vi "保存程序.vi"(8 "error in (no error)":errorcluster caption="错误输入（无错误）", 11 "程序 输入":refnum<class "程序.lvclass">) -> (0 "error out":errorcluster caption="错误输出", 3 "程序 输出":refnum<class "程序.lvclass">)   [LabVIEW 2020, in "程序.lvclass"]
uses:
  D:/SuperPython-master/ScintillaNET.dll
  ScintillaNET.dll
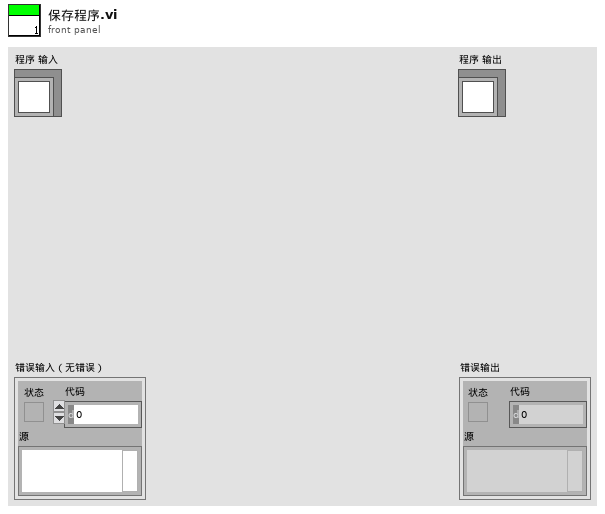
[diagram p1: front panel]
types:
  T1 = enum16{"open", "replace", "create", "open or create", "replace or create", "replace or create with confirmation"}
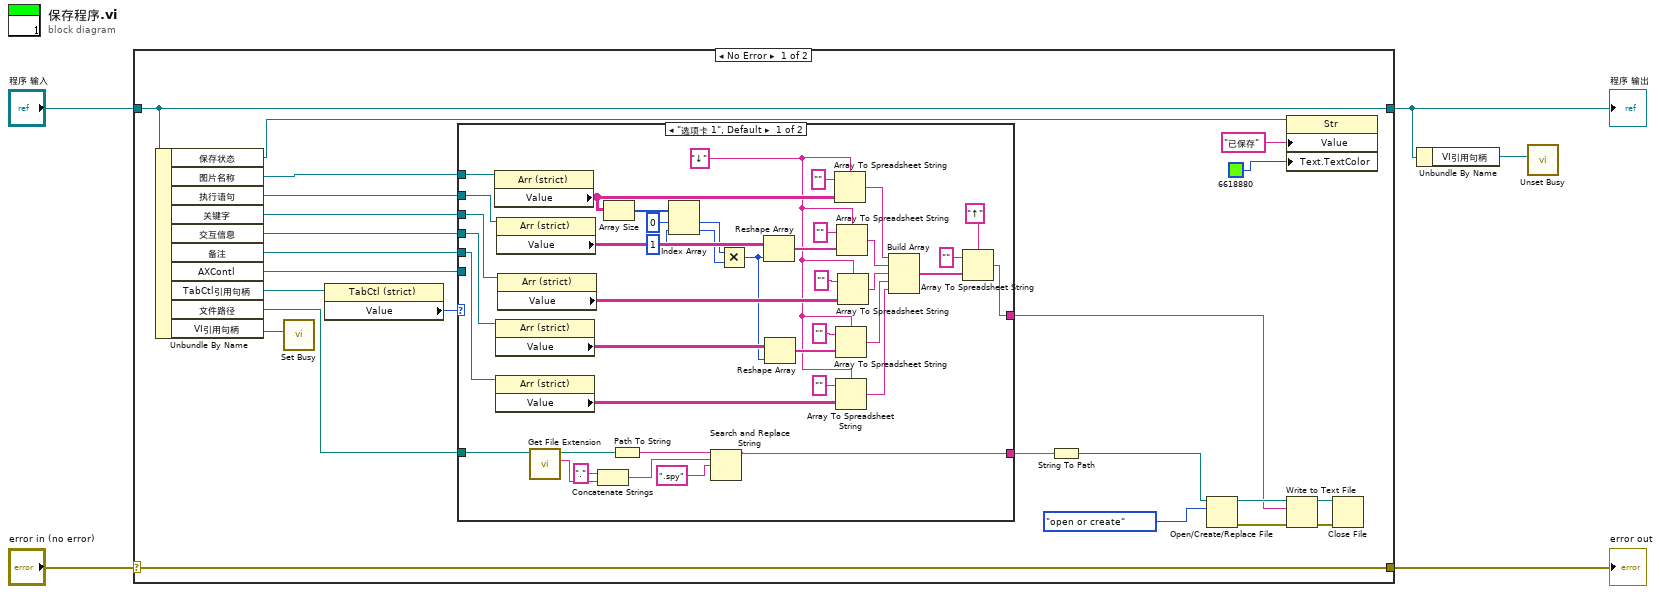
[diagram p0: block diagram]
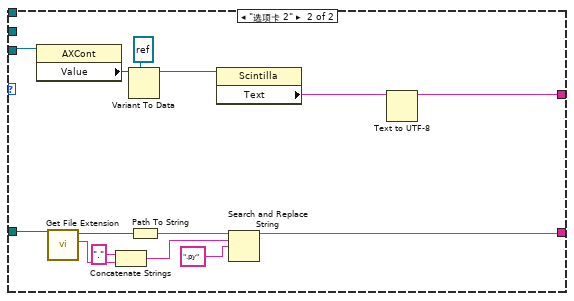
[diagram p2: hidden frame]
diagram:
  n1 = case shown="No Error" "error in (no error)" {
    selector: "error in (no error)" -> [w28 w85]
    tunnel: [w28 w85] -> w4
    tunnel: [w22 w84] -> w2
    tunnel: "程序 输入" -> [w22 w84]
    frame No Error {
      n2 = Unbundle By Name(w22) -> ("保存状态"=w14:refnum<vi>, "图片名称"=w21:refnum<vi>, "执行语句"=w20:refnum<vi>, "关键字"=w19:refnum<vi>, "交互信息"=w17:refnum<vi>, "备注"=w16:refnum<vi>, "AXContl"=w11:refnum<vi>, "TabCtl引用句柄"=w10:refnum<vi>, "文件路径"=w8:path, "VI引用句柄"=w12:refnum<vi>)
      n3 = call <vilib>:"Set Busy.vi"("VI reference (current VI)"=w12) -> ()  [unwired: 9 in, 2 out]
      n4 = property class="TabCtl (strict)"(reference=w10) -> ("Value"=w9:enum32{"选项卡 1", "选项卡 2"})  [unwired: 1 in, 2 out]
      n5 = case shown="\"选项卡 1\", Default" w9 {
        tunnel: [w68 w70] -> w23
        tunnel: w21 -> [w66 _]
        tunnel: w20 -> [w65 _]
        tunnel: w19 -> [w64 _]
        tunnel: w17 -> [w54 _]
        tunnel: w16 -> [w41 _]
        tunnel: w11 -> [_ w80]
        tunnel: w8 -> [w30 w79]
        tunnel: [w29 w73] -> w7
        frame "选项卡 1", Default {
          w38 = "↓" ("分隔符(Tab)")
          n6 = property class="Arr (strict)"(reference=w66) -> ("Value"=w48:string[][])  [unwired: 1 in, 2 out]
          n7 = property class="Arr (strict)"(reference=w54) -> ("Value"=w52:string[][])  [unwired: 1 in, 2 out]
          n8 = property class="Arr (strict)"(reference=w41) -> ("Value"=w40:string[][])  [unwired: 1 in, 2 out]
          n9 = property class="Arr (strict)"(reference=w65) -> ("Value"=w50:string[][])  [unwired: 1 in, 2 out]
          n10 = property class="Arr (strict)"(reference=w64) -> ("Value"=w60:string[][])  [unwired: 1 in, 2 out]
          n11 = call <vilib>:"Get File Extension.vi"("file"=w30) -> ("lowercase file extension"=w33:string, "dup file"=w36:path)  [unwired: 6 in, 3 out]
          n12 = Concatenate Strings("." ("字符串"), w33) -> (w32:string)
          n13 = Array Size(array=w48) -> (size(s)=w47:i32[])
          n14 = Path To String(path=w36) -> (string=w35:string)
          n15 = Index Array(array=w47, index #1=0 ("索引"), index #2=1 ("索引")) -> (element #1=w44:i32, element #2=w43:i32)
          n16 = Search and Replace String(input string=w35, search string=w32, replace string=".spy" ("字符串")) -> (result string=w29:string)  [unwired: 5 in, 3 out]
          n17 = Multiply(x=w44, y=w43) -> (x*y=w42:i32)
          n18 = Reshape Array(w50, w42) -> (w49:string[])
          n19 = Reshape Array(w52, w42) -> (w51:string[])
          n20 = Array To Spreadsheet String(delimiter (Tab)=w38, array=w48, 3:"" ("格式字符串")) -> (spreadsheet string=w59:string)
          n21 = Array To Spreadsheet String(delimiter (Tab)=w38, array=w51, 3:"" ("格式字符串")) -> (spreadsheet string=w53:string)
          n22 = Array To Spreadsheet String(delimiter (Tab)=w38, array=w40, 3:"" ("格式字符串")) -> (spreadsheet string=w37:string)
          n23 = Array To Spreadsheet String(delimiter (Tab)=w38, array=w49, 3:"" ("格式字符串")) -> (spreadsheet string=w58:string)
          n24 = Array To Spreadsheet String(delimiter (Tab)=w38, array=w60, 3:"" ("格式字符串")) -> (spreadsheet string=w57:string)
          n25 = Build Array(w59, w58, w57, w53, w37) -> (w56:string[])
          n26 = Array To Spreadsheet String(delimiter (Tab)="↑" ("分隔符(Tab)"), array=w56, 3:"" ("格式字符串")) -> (spreadsheet string=w68:string)
        }
        frame "选项卡 2" {
          n27 = property class="AXCont"(reference=w80) -> ("Value"=w81:variant)  [unwired: 1 in, 2 out]
          n28 = call <vilib>:"Get File Extension.vi"("file"=w79) -> ("lowercase file extension"=w75:string, "dup file"=w78:path)  [unwired: 6 in, 3 out]
          n29 = Concatenate Strings("." ("字符串"), w75) -> (w74:string)
          n30 = Variant To Data(type=refnum<k24> refnum ("文本编辑"), Variant=w81) -> (data=w82:refnum<k24>)  [unwired: 1 in, 1 out]
          n31 = Path To String(path=w78) -> (string=w77:string)
          n32 = property class="Scintilla"(reference=w82) -> ("Text"=w71:string)  [unwired: 1 in, 2 out]
          n33 = Search and Replace String(input string=w77, search string=w74, replace string=".py" ("字符串")) -> (result string=w73:string)  [unwired: 5 in, 3 out]
          n34 = Text to UTF-8 ("文本至UTF-8转换")(11:w71) -> (3:w70:string)  [unwired: 2 in, 1 out]
        }
      }
      n35 = String To Path(string=w7) -> (path=w6:path)
      n36 = Open/Create/Replace File(file path (use dialog)=w6, operation (0:open)=T1."open or create" ("操作(0:open)")) -> (refnum out=w27:refnum<file>, error out=w26:errorcluster)  [unwired: 4 in, 1 out]
      n37 = property class="Str"(reference=w14, "Value"="已保存" ("值"), "Text.TextColor"=u32 6618880) -> ()  [unwired: 1 in, 2 out]
      n38 = Write to Text File(file (use dialog)=w27, text=w23, error in=w26) -> (refnum out=w25:refnum<file>, error out=w24:errorcluster)  [unwired: 1 in, 1 out]
      n39 = Close File(refnum=w25, error in=w24) -> ()  [unwired: 2 out]
    }
    frame Error {
    }
  }
  "error out" <- w4
  "程序 输出" <- w2
  n40 = Unbundle By Name(w2) -> ("VI引用句柄"=w1:refnum<vi>)
  n41 = call <vilib>:"Unset Busy.vi"("VI reference (current VI)"=w1) -> ()  [unwired: 10 in, 1 out]
